vi "Draw BMP at Location.vi"(6 "top":i16=200, 9 "left":i16=200, 10 "selected path":path, 11 "picture in":picture) -> (1 "Thumbnail":T1, 2 "image data":T2, 3 "picture out":picture)   [LabVIEW 2018]
uses:
  <vilib>/picture/picture.llb/imagedata.ctl
  Thumbnail Cluster.ctl
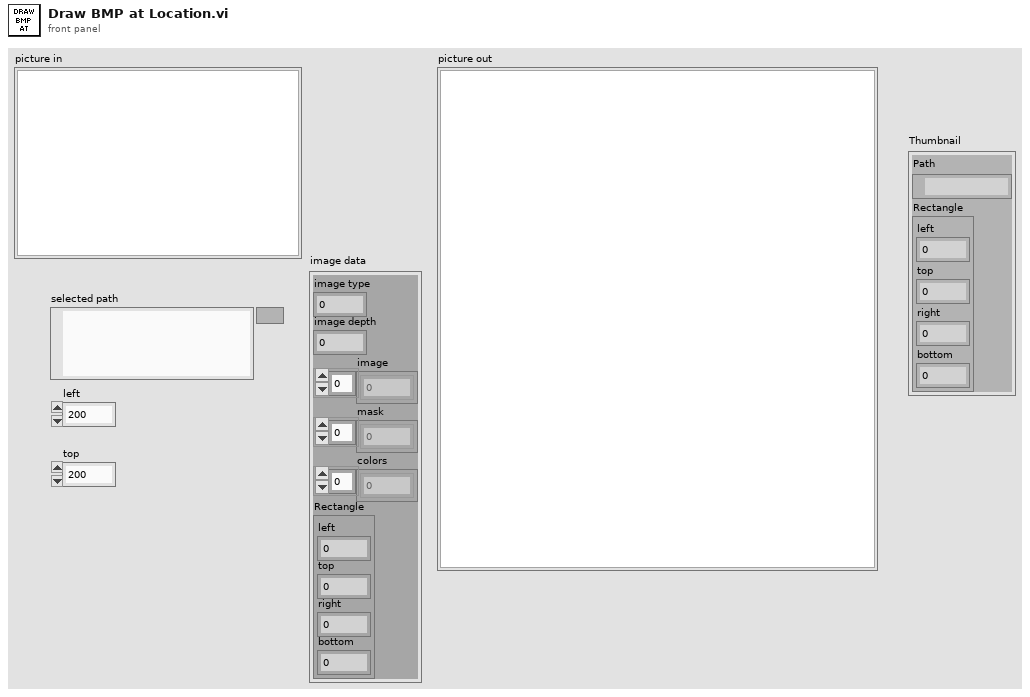
[diagram p1: front panel]
types:
  T1 = typedef "Thumbnail Cluster.ctl" = cluster{"Path":path, "Rectangle":cluster{"left":i16, "top":i16, "right":i16, "bottom":i16}}
  T2 = typedef "imagedata.ctl" = cluster{"image type":i32, "image depth":i32, "image":u8[], "mask":u8[], "colors":u32[], "Rectangle":cluster{"left":i16, "top":i16, "right":i16, "bottom":i16}}
  T3 = cluster{"left":i16, "top":i16, "right":i16, "bottom":i16}
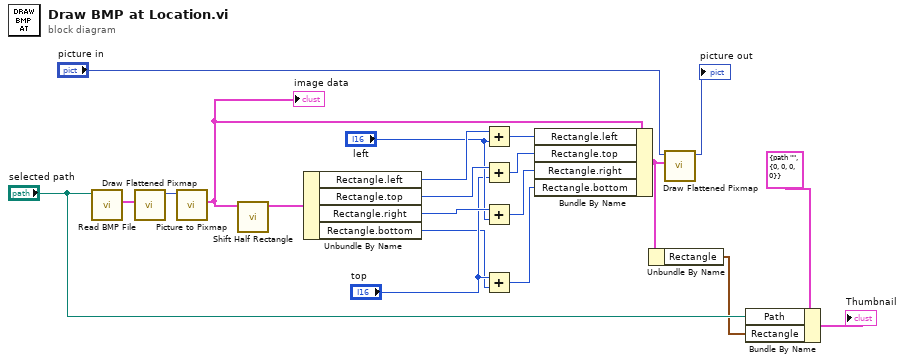
[diagram p0: block diagram]
diagram:
  n1 = call <vilib>:"Read BMP File.vi"("path to BMP file"="selected path") -> ("image data"=w18:T2)  [unwired: 8 in, 2 out]
  n2 = call <vilib>:"Draw Flattened Pixmap.vi"("image data"=w18) -> ("new picture"=w19:picture)  [unwired: 8 in]
  n3 = call <vilib>:"Picture to Pixmap.vi"("picture"=w19) -> ("image data"=w2:T2)  [unwired: 9 in, 1 out]
  "image data" <- w2
  n4 = call "Shift Half Rectangle.vi"("image data in"=w2) -> ("image data out"=w1:T2)  [unwired: 10 in]
  n5 = Unbundle By Name(w1) -> ("Rectangle.left"=w17:i16, "Rectangle.top"=w15:i16, "Rectangle.right"=w13:i16, "Rectangle.bottom"=w9:i16)
  n6 = Add(x=w17, y="left") -> (x+y=w16:i16)
  n7 = Add(x=w15, y="top") -> (x+y=w14:i16)
  n8 = Add(x=w13, y="left") -> (x+y=w11:i16)
  n9 = Add(x="top", y=w9) -> (x+y=w8:i16)
  n10 = Bundle By Name(cluster=w2, "Rectangle.left"=w16, "Rectangle.top"=w14, "Rectangle.right"=w11, "Rectangle.bottom"=w8) -> (w7:T2)
  n11 = Unbundle By Name(w7) -> ("Rectangle"=w3:T3)
  n12 = call <vilib>:"Draw Flattened Pixmap.vi"("image data"=w7, "picture"="picture in") -> ("new picture"=→"picture out":picture)  [unwired: 7 in]
  n13 = Bundle By Name(cluster=T1 {"Path"=path "", "Rectangle"={"left"=0, "top"=0, "right"=0, "bottom"=0}} ("Thumbnail"), "Path"="selected path", "Rectangle"=w3) -> (→"Thumbnail":T1)
